vi "Replace Engine Project Content.vi"(7 "CDFolderPath String":string, 8 "error in":errorcluster, 9 "Custom Device Project Path":path, 10 "CD Name":string, 11 "Template Project path":path) -> (0 "error out":errorcluster)   [LabVIEW 2026, in "NIVS_CDEW_MetaDataObj.lvclass"]
uses:
  NIVS_CDEW_MetaDataObj.lvclass
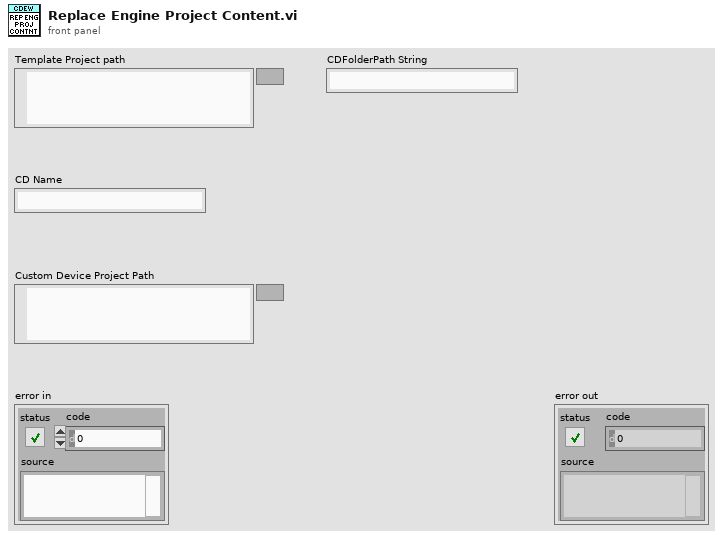
[diagram p1: front panel]
types:
  T1 = enum16{"open", "replace", "create", "open or create", "replace or create", "replace or create with confirmation"}
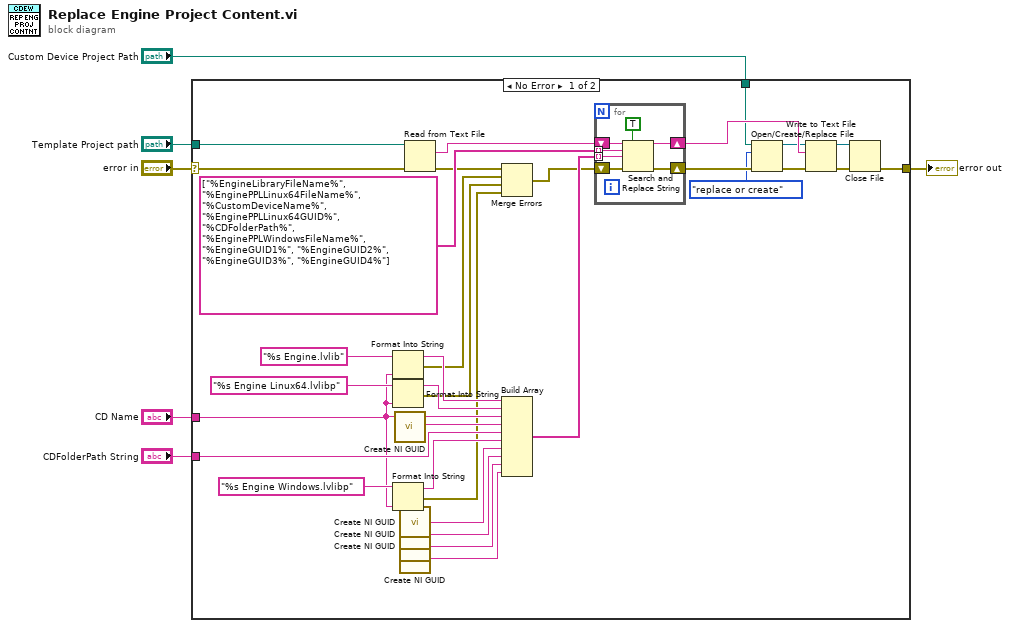
[diagram p0: block diagram]
diagram:
  n1 = case shown="No Error" "error in" {
    selector: "error in" -> [w22 w46]
    tunnel: "Template Project path" -> [w38 _]
    tunnel: [w35 w46] -> w5
    tunnel: "Custom Device Project Path" -> [w27 _]
    tunnel: "CD Name" -> [w17 _]
    tunnel: "CDFolderPath String" -> [w19 _]
    frame No Error {
      n2 = Format Into String(format string="%s Engine.lvlib", w17) -> (resulting string=w31:string, error out=w13:errorcluster)  [unwired: 2 in]
      n3 = Format Into String(format string="%s Engine Linux64.lvlibp", w17) -> (resulting string=w32:string, error out=w12:errorcluster)  [unwired: 2 in]
      n4 = Format Into String(format string="%s Engine Windows.lvlibp", w17) -> (resulting string=w16:string, error out=w11:errorcluster)  [unwired: 2 in]
      n5 = call <vilib>:"Create NI GUID.vi"() -> ("NI GUID"=w21:string)
      n6 = call <vilib>:"Create NI GUID.vi"() -> ("NI GUID"=w15:string)
      n7 = call <vilib>:"Create NI GUID.vi"() -> ("NI GUID"=w9:string)
      n8 = call <vilib>:"Create NI GUID.vi"() -> ("NI GUID"=w8:string)
      n9 = call <vilib>:"Create NI GUID.vi"() -> ("NI GUID"=w7:string)
      n10 = Read from Text File(file (use dialog)=w38, error in=w22) -> (text=w34:string, error out=w14:errorcluster)  [unwired: 2 in, 2 out]
      n11 = Merge Errors(w14, w13, w12, w11) -> (w10:errorcluster)
      n12 = Build Array(w31, w32, w17, w21, w19, w16, w15, w9, w8, w7) -> (w29:string[])
      n13 = for {
        shift-right: [w44] -> w37
        shift-left: w10 -> [w43]
        shift-right: [w39] -> w28
        shift-left: w34 -> [w42]
        tunnel: string[] ["%EngineLibraryFileName%", "%EnginePPLLinux64FileName%", "%CustomDeviceName%", "%EnginePPLLinux64GUID%", "%CDFolderPath%", "%EnginePPLWindowsFileName%", "%EngineGUID1%", "%EngineGUID2%", "%EngineGUID3%", "%EngineGUID4%"] -> [w41] mode=indexing
        tunnel: w29 -> [w40] mode=indexing
        n14 = Search and Replace String(replace all?=TRUE ("replace all? (F)"), input string=w42, search string=w41, replace string=w40, error in=w43) -> (result string=w39:string, error out=w44:errorcluster)  [unwired: 3 in, 2 out]
      }
      n15 = Open/Create/Replace File(file path (use dialog)=w27, error in=w37, operation (0:open)=T1."replace or create") -> (refnum out=w26:refnum<file>, error out=w25:errorcluster)  [unwired: 3 in, 1 out]
      n16 = Write to Text File(file (use dialog)=w26, text=w28, error in=w25) -> (refnum out=w24:refnum<file>, error out=w23:errorcluster)  [unwired: 1 in, 1 out]
      n17 = Close File(refnum=w24, error in=w23) -> (error out=w35:errorcluster)  [unwired: 1 out]
    }
    frame Error {
    }
  }
  "error out" <- w5
